vi "PIP_to_TXT.vi"(8 "error in":errorcluster) -> (0 "error out":errorcluster, 2 "FileName":string)   [LabVIEW 2018]
uses:
  Global Variables.vi
panel:
  out "PIP_to_JSN":string[](array[string])
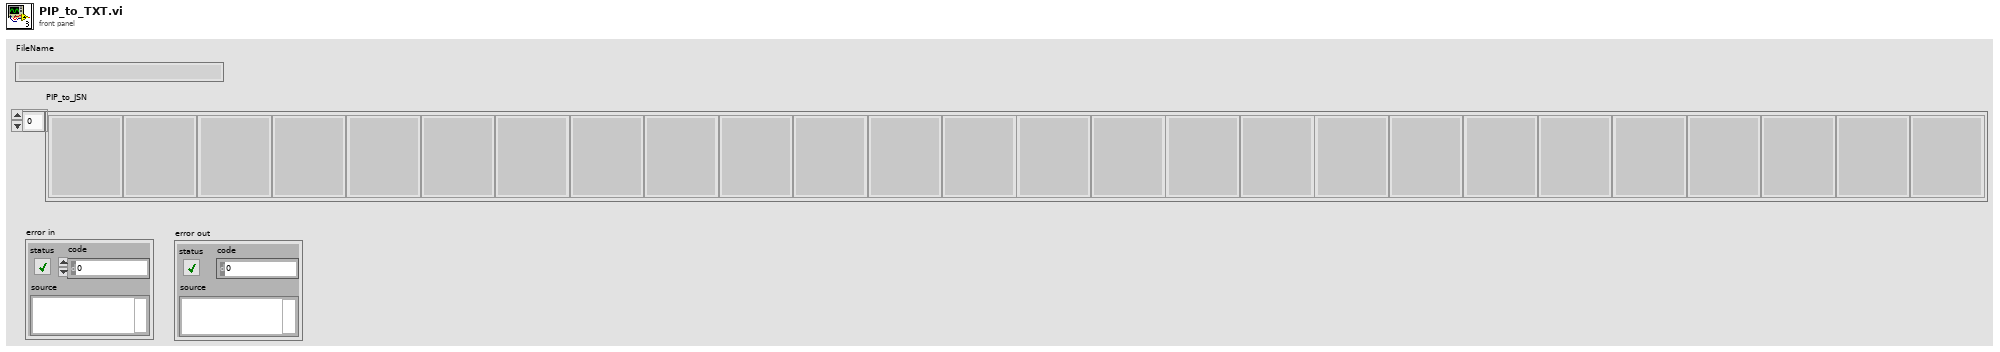
[diagram p1: front panel]
types:
  T1 = enum16{"open", "replace", "create", "open or create", "replace or create", "replace or create with confirmation"}
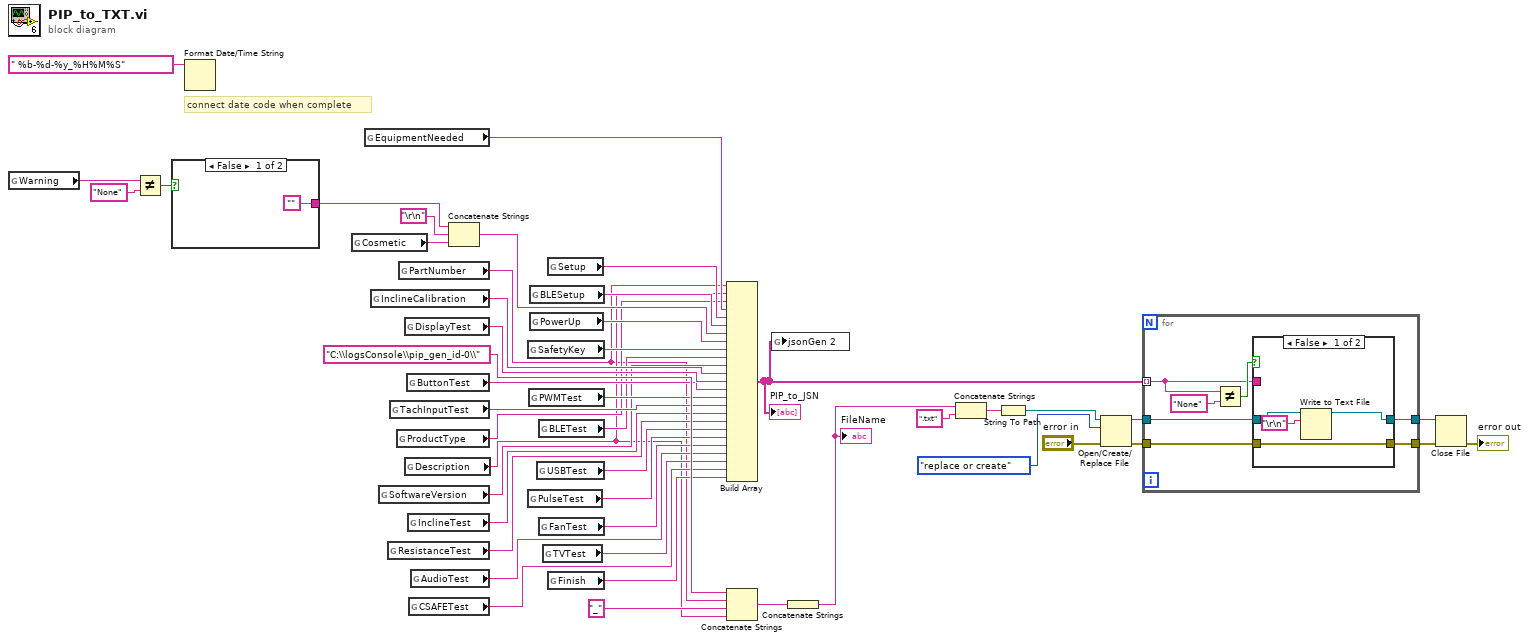
[diagram p0: block diagram]
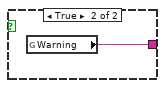
[diagram p2: hidden frame]
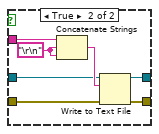
[diagram p3: hidden frame]
diagram:
  # "connect date code when complete"
  n1 = global read "Global Variables.vi" "Warning"() -> (w4:string)
  n2 = Not Equal?(x=w4, y="None") -> (x != y?=w5:bool)
  n3 = case shown="False" w5 {
    tunnel: ["" w49] -> w2
    frame False {
    }
    frame True {
      n4 = global read "Global Variables.vi" "Warning"() -> (w49:string)
    }
  }
  n5 = Format Date/Time String(time format string (%c)=" %b-%d-%y_%H%M%S") -> ()  [unwired: 2 in, 1 out]
  n6 = global read "Global Variables.vi" "Cosmetic"() -> (w41:string)
  n7 = global read "Global Variables.vi" "EquipmentNeeded"() -> (w11:string)
  n8 = global read "Global Variables.vi" "InclineCalibration"() -> (w39:string)
  n9 = global read "Global Variables.vi" "SoftwareVersion"() -> (w18:string)
  n10 = global read "Global Variables.vi" "ResistanceTest"() -> (w33:string)
  n11 = global read "Global Variables.vi" "TachInputTest"() -> (w35:string)
  n12 = global read "Global Variables.vi" "ProductType"() -> (w10:string)
  n13 = global read "Global Variables.vi" "PartNumber"() -> (w8:string)
  n14 = global read "Global Variables.vi" "DisplayTest"() -> (w38:string)
  n15 = global read "Global Variables.vi" "Description"() -> (w9:string)
  n16 = global read "Global Variables.vi" "ButtonTest"() -> (w37:string)
  n17 = global read "Global Variables.vi" "InclineTest"() -> (w34:string)
  n18 = global read "Global Variables.vi" "CSAFETest"() -> (w27:string)
  n19 = global read "Global Variables.vi" "AudioTest"() -> (w29:string)
  n20 = Concatenate Strings(w2, "\r\n", w41) -> (w14:string)
  n21 = global read "Global Variables.vi" "SafetyKey"() -> (w16:string)
  n22 = global read "Global Variables.vi" "PulseTest"() -> (w31:string)
  n23 = global read "Global Variables.vi" "PWMTest"() -> (w36:string)
  n24 = global read "Global Variables.vi" "BLESetup"() -> (w13:string)
  n25 = global read "Global Variables.vi" "PowerUp"() -> (w15:string)
  n26 = global read "Global Variables.vi" "USBTest"() -> (w32:string)
  n27 = global read "Global Variables.vi" "BLETest"() -> (w17:string)
  n28 = global read "Global Variables.vi" "FanTest"() -> (w30:string)
  n29 = global read "Global Variables.vi" "TVTest"() -> (w28:string)
  n30 = global read "Global Variables.vi" "Setup"() -> (w12:string)
  n31 = global read "Global Variables.vi" "Finish"() -> (w26:string)
  n32 = Build Array(w8, w9, w10, w11, w12, w13, w14, w15, w16, w17, w18, w39, w38, w37, w36, w35, w34, w33, w32, w31, w30, w29, w28, w27, w26) -> (w1:string[])
  "PIP_to_JSN" <- w1
  n33 = Concatenate Strings("C:\\logsConsole\\pip_gen_id-0\\" ("Path"), w8, "_" ("string"), w9) -> (w22:string)
  n34 = global write "Global Variables.vi" "jsonGen 2"(w1) -> ()
  n35 = Concatenate Strings(w22) -> (w20:string)
  "FileName" <- w20
  n36 = Concatenate Strings(w20, ".txt") -> (w21:string)
  n37 = String To Path(string=w21) -> (path=w42:path)
  n38 = Open/Create/Replace File(file path (use dialog)=w42, error in="error in", operation (0:open)=T1."replace or create") -> (refnum out=w47:refnum<file>, error out=w46:errorcluster)  [unwired: 3 in, 1 out]
  n39 = for {
    tunnel: w46 -> [w53]
    tunnel: w47 -> [w54]
    tunnel: w1 -> [w50] mode=indexing
    tunnel: [w52] -> w7
    tunnel: [w51] -> w6
    n40 = Not Equal?(x=w50, y="None") -> (x != y?=w56:bool)
    n41 = case shown="False" w56 {
      tunnel: w50 -> [_ w64]
      tunnel: [w60 w65] -> w51
      tunnel: w54 -> [w58 w63]
      tunnel: w53 -> [w57 w62]
      tunnel: [w57 w61] -> w52
      frame False {
        n42 = Write to Text File(file (use dialog)=w58, text="\r\n") -> (refnum out=w60:refnum<file>)  [unwired: 2 in, 2 out]
      }
      frame True {
        w67 = "\r\n"
        n43 = Concatenate Strings(w64, w67, w67) -> (w66:string)
        n44 = Write to Text File(file (use dialog)=w63, text=w66, error in=w62) -> (refnum out=w65:refnum<file>, error out=w61:errorcluster)  [unwired: 1 in, 1 out]
      }
    }
  }
  n45 = Close File(refnum=w6, error in=w7) -> (error out=→"error out":errorcluster)  [unwired: 1 out]
